vi "Marker Draw and Commands Loop.vi"(4 "Cursor Options":T1={"font"={"Font Name"="Arial", "Size"=15, "Strikeout?"=FALSE, "Italic?"=FALSE, "Underline?"=FALSE, "Outline?"=FALSE, "Shadow?"=FALSE, "Bold?"=FALSE}, "size"=2, "Timestamp"=enum."at BOTTOM", "Vertical Line?"=TRUE, "Horizontal Line?"=TRUE, "alignment(left, top)"={"horizontal"=enum."left", "vertical"=enum."center"}, "TextFormat"=" %3$s\\n %2$.2f", "time format (%H:%M:%S)"="%I:%M:%S %p"} {"size" min=1 max=50}, 6 "Enable Cursors":bool, 9 "Markers":T2[](array[typedef]), 10 "XY Graph":refnum<vi>, 11 "Options":T4={"Color"=16723218, "pen"={"Width"=2, "Style"=enum."Solid"}, "font"={"Font Name"="Arial", "Size"=14, "Strikeout?"=FALSE, "Italic?"=FALSE, "Underline?"=FALSE, "Outline?"=FALSE, "Shadow?"=FALSE, "Bold?"=FALSE, "FontColor"=6908265}, "caption"="Click to set a point marker"}) -> ()   [LabVIEW 2014, in "Graph Extensions.lvlib"]
doc: "This draw loop is the command processor thread and redraw thread to handle the events from the UI. It can be started anywhere with a reference to the graph. Markers work only when the graph palette tool is in cursor mode, as it replaces that mode since Graph extensions have their own improved cursors/markers, that mode is not needed. \n\n<B>Options</B> can be changed by the user using the right click menu with the markers.\n<B>Markers</B> input can be used to initialize a known set of markers (eitehr loaded from disk or programmatically created)\n\n<B>Cursers Enabled</B> activates the other graph extension (cursors) when usual mouse move occurs."
uses:
  Graph Extensions.lvlib
  controls/MarkerInfo.ctl
  <vilib>/Utility/miscctls.llb/LVPoint32TypeDef.ctl
  controls/markerType.ctl
  controls/commands.ctl
  controls/GraphExt-Cmds.ctl
  controls/cmd_options.ctl
  controls/Simple Global for Marker Options.vi
  controls/MarkerOptions.ctl
  controls/CursorOptions.ctl
panel:
  in  "stop":bool
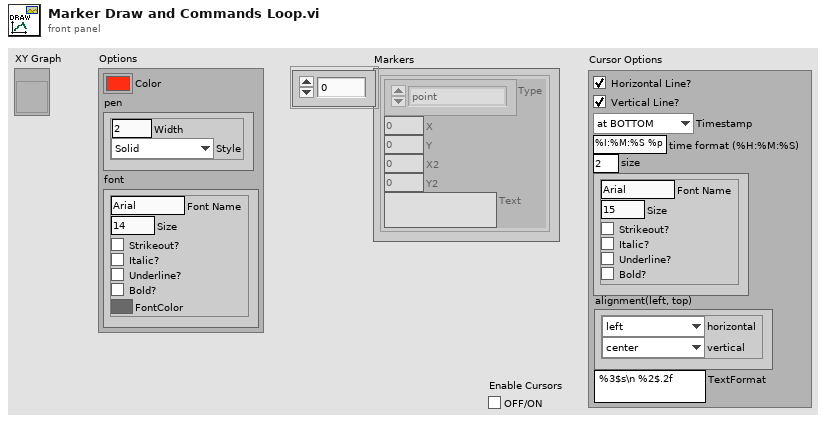
[diagram p1: front panel]
types:
  T1 = typedef "Graph Extensions.lvlib/CursorOptions.ctl" = cluster{"font":cluster{"Font Name":string, "Size":i16, "Strikeout?":bool, "Italic?":bool, "Underline?":bool, "Outline?":bool, "Shadow?":bool, "Bold?":bool}, "size":i16, "Timestamp":enum16{"at TOP", "at BOTTOM", "none"}, "Vertical Line?":bool, "Horizontal Line?":bool, "alignment(left, top)":cluster{"horizontal":enum16{"left", "center", "right"}, "vertical":enum16{"top", "center", "bottom"}}, "TextFormat":string, "time format (%H:%M:%S)":string}
  T2 = typedef "Graph Extensions.lvlib/MarkerInfo.ctl" = cluster{"Type":T3, "X":dbl, "Y":dbl, "X2":dbl, "Y2":dbl, "Text":string}
  T3 = typedef "Graph Extensions.lvlib/markerType.ctl" = enum16{"point", "arrow", "horiz", "vert", "vert range", "horiz range", "box"}
  T4 = typedef "Graph Extensions.lvlib/MarkerOptions.ctl" = cluster{"Color":u32, "pen":cluster{"Width":u16, "Style":enum32{"Solid", "Dash", "Dot", "DashDot", "DashDotDot"}}, "font":cluster{"Font Name":string, "Size":i16, "Strikeout?":bool, "Italic?":bool, "Underline?":bool, "Outline?":bool, "Shadow?":bool, "Bold?":bool, "FontColor":u32}, "caption":string}
  T5 = typedef "Graph Extensions.lvlib/commands.ctl" = enum16{"up", "options", "click", "move", "type", "redraw", "edited", "exit"}
  T6 = typedef "LVPoint32TypeDef.ctl" = cluster{"Horizontal":i32, "Vertical":i32}
  T7 = cluster{"cmd":T5, "Type":T3, "Coords":T6, "Active Tool":i32, "mode":enum16{"drag", "none"}}
  T8 = typedef "Graph Extensions.lvlib/GraphExt-Cmds.ctl" = cluster{"cmd":T5, "Type":T3, "Coords":T6, "text":string}
  T9 = typedef "Graph Extensions.lvlib/cmd_options.ctl" = cluster{"Marker Color":u32, "Style":enum32{"Solid", "Dash", "Dot", "DashDot", "DashDotDot"}, "Width":u16, "Size":i16, "Color":u32}
  T10 = typedef "LVRectTypeDef.ctl" = cluster{"Left":i16, "Top":i16, "Right":i16, "Bottom":i16}
  T11 = enum32{"Solid", "Dash", "Dot", "DashDot", "DashDotDot"}
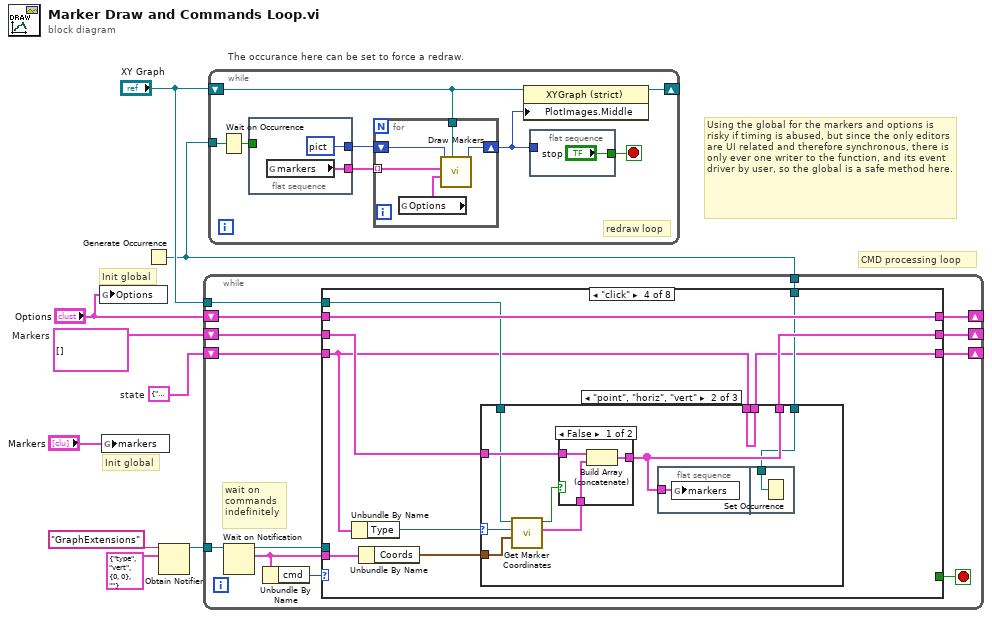
[diagram p0: block diagram]
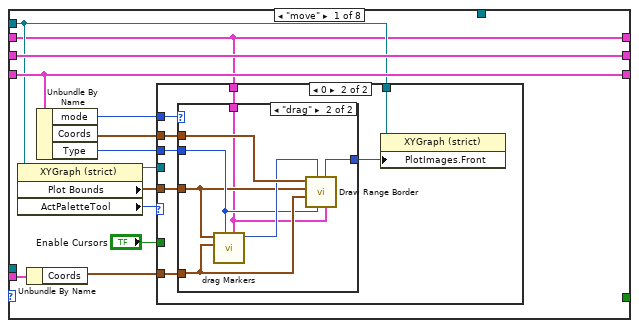
[diagram p2: hidden frame]
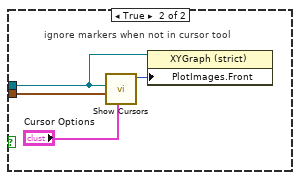
[diagram p4: hidden frame]
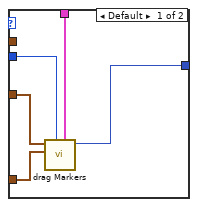
[diagram p5: hidden frame]
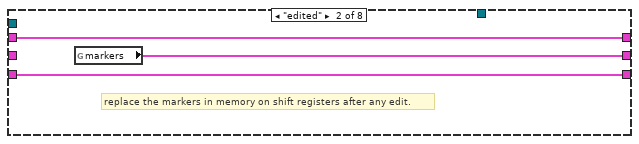
[diagram p6: hidden frame]
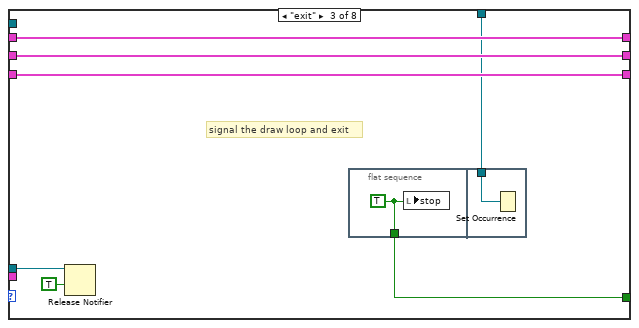
[diagram p7: hidden frame]
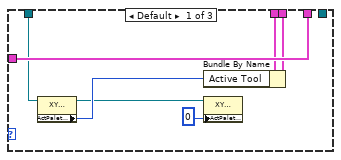
[diagram p8: hidden frame]
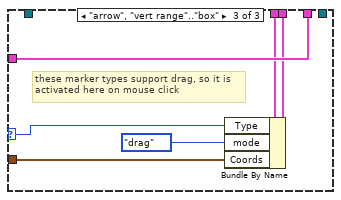
[diagram p10: hidden frame]
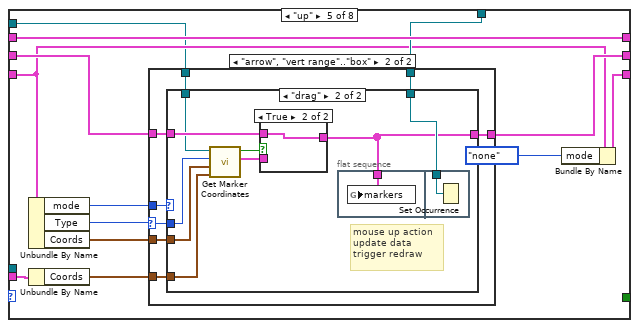
[diagram p11: hidden frame]
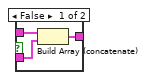
[diagram p14: hidden frame]
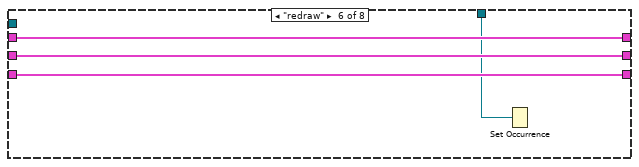
[diagram p15: hidden frame]
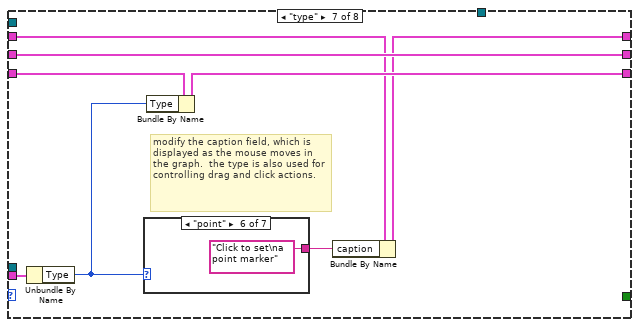
[diagram p16: hidden frame]
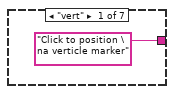
[diagram p17: hidden frame]
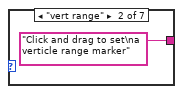
[diagram p18: hidden frame]
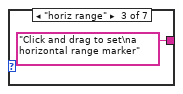
[diagram p19: hidden frame]
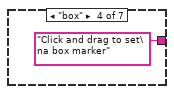
[diagram p20: hidden frame]
diagram:
  w5 = T7 {"cmd"=enum."click", "Type"=enum."point", "Coords"={"Horizontal"=0, "Vertical"=0}, "Active Tool"=0, "mode"=enum."none"}  # state
  w4 = T2[] []  # Markers
  # "Init global"
  # "CMD processing loop"
  # "Using the global for the markers and options is risky if timing is abused, but since the only editors are UI related and therefore synchronous, there is only ever one writer to the function, and its event driver by user, so the global is a safe method here."
  # "Init global"
  # "The occurance here can be set to force a redraw."
  n1 = global write "Simple Global for Marker Options.vi" "Options"("Options") -> ()
  n2 = global write "Simple Global for Marker Options.vi" "markers"("Markers") -> ()
  n3 = Generate Occurrence() -> (w3:refnum<k4>)
  n4 = Obtain Notifier(name (unnamed)="GraphExtensions", notification data type=T8 {"cmd"=enum."type", "Type"=enum."vert", "Coords"={"Horizontal"=0, "Vertical"=0}, "text"=""}) -> (notifier out=w8:refnum<notifier>)  [unwired: 2 in, 2 out]
  n5 = while {
    tunnel: w8 -> [w22]
    shift-right: [w18] -> _
    shift-left: "Options" -> [w19]
    shift-right: [w17] -> _
    shift-left: w4 -> [w16]
    shift-right: [w15] -> _
    shift-left: w5 -> [w14]
    tunnel: w3 -> [w13]
    tunnel: "XY Graph" -> [w12]
    stop <- w11 stop-if-true
    # "wait on\ncommands\nindefinitely"
    n6 = Wait on Notification(notifier=w22) -> (notifier out=w10:refnum<notifier>, notification=w21:T8)  [unwired: 3 in, 2 out]
    n7 = Unbundle By Name(w21) -> ("cmd"=w20:T5)
    n8 = case shown="\"click\"" w20 {
      tunnel: w19 -> [w26 w65 w72 w84 w125 w152 w156 w176]
      tunnel: w21 -> [w35 _ _ w83 w124 _ w161 w181]
      tunnel: [w26 w65 w72 w84 w125 w152 w155 w171] -> w18
      tunnel: [w34 w63 w71 w82 w118 w154 w162 w183] -> w17
      tunnel: w16 -> [w34 _ w71 w78 w119 w154 w162 w183]
      tunnel: [w33 w64 w70 w79 w115 w153 w159 w182] -> w15
      tunnel: w14 -> [w33 w64 w70 w77 w116 w153 w160 w182]
      tunnel: w13 -> [_ _ w68 w81 w117 w151 _ w170]
      tunnel: w12 -> [w28 _ _ w80 w113 _ _ _]
      tunnel: [_ _ w69 _ _ _ _ _] -> w11
      tunnel: w10 -> [_ _ w67 _ _ _ _ _]
      frame "move" {
        n9 = property on="Property Node" class="XYGraph (strict)"(reference=w28) -> (reference out=w24:refnum<vi>, "Plot Bounds"=w27:T10, "ActPaletteTool"=w25:i32)  [unwired: 1 in, 1 out]
        n10 = Unbundle By Name(w35) -> ("Coords"=w29:T6)
        n11 = Unbundle By Name(w33) -> ("mode"=w31:enum16{"drag", "none"}, "Coords"=w32:T6, "Type"=w30:T3)
        n12 = case shown="0" w25 {
          tunnel: w32 -> [_ w50]
          tunnel: w31 -> [_ w48]
          tunnel: w30 -> [_ w47]
          tunnel: w29 -> [w37 w46]
          tunnel: w28 -> [_ w45]
          tunnel: w27 -> [_ w44]
          tunnel: w26 -> [_ w43]
          tunnel: w24 -> [w38 _]
          tunnel: "Enable Cursors" -> [w36 _]
          frame Default {
            n13 = case shown="False" w36 {
              tunnel: w38 -> [_ w40]
              tunnel: w37 -> [_ w39]
              frame False {
              }
              frame True {
                # "ignore markers when not in cursor tool"
                n14 = call "Show Cursors.vi"("Cursor Options"="Cursor Options", "Coords"=w39, "XY Graph"=w40) -> ("output picture"=w42:picture)  [unwired: 7 in, 1 out]
                n15 = property on="Property Node" class="XYGraph (strict)"(reference=w40, "PlotImages.Front"=w42) -> ()  [unwired: 1 in, 2 out]
              }
            }
          }
          frame 0 {
            n16 = case shown="\"drag\"" w48 {
              tunnel: w50 -> [_ w62]
              tunnel: [w55 w61] -> w49
              tunnel: w43 -> [w54 w56]
              tunnel: w47 -> [w53 w58]
              tunnel: w46 -> [w52 w59]
              tunnel: w44 -> [w51 w57]
              frame Default {
                n17 = call "drag Markers.vi"("Marker Options"=w54, "Type"=w53, "Coords"=w52, "Plot Area Bounds"=w51) -> ("new picture"=w55:picture)  [unwired: 7 in]
              }
              frame "drag" {
                n18 = call "drag Markers.vi"("Marker Options"=w56, "Type"=w58, "Coords"=w59, "Plot Area Bounds"=w57) -> ("new picture"=w60:picture)  [unwired: 7 in]
                n19 = call "Draw Range Border.vi"("Marker Options"=w56, "Type"=w58, "picture"=w60, "end Coords"=w59, "Plot Bounds"=w57, "Start Coords"=w62) -> ("new picture"=w61:picture)  [unwired: 5 in]
              }
            }
            n20 = property on="Property Node" class="XYGraph (strict)"(reference=w45, "PlotImages.Front"=w49) -> ()  [unwired: 1 in, 2 out]
          }
        }
      }
      frame "edited" {
        # "replace the markers in memory on shift registers after any edit."
        n21 = global read "Simple Global for Marker Options.vi" "markers"() -> (w63:T2[])
      }
      frame "exit" {
        # "signal the draw loop and exit"
        n22 = Release Notifier(notifier=w67, force destroy? (F)=TRUE) -> ()  [unwired: 1 in, 3 out]
        n23 = flat-sequence {
          tunnel: [w73] -> w69
          tunnel: w68 -> [w74]
          frame #0 {
            w73 = TRUE
            n24 = local write "stop"(w73) -> ()
          }
          frame #1 {
            n25 = Set Occurrence(w74) -> ()
          }
        }
      }
      frame "click" {
        n26 = Unbundle By Name(w77) -> ("Type"=w76:T3)
        n27 = Unbundle By Name(w83) -> ("Coords"=w75:T6)
        n28 = case shown="\"point\", \"horiz\", \"vert\"" w76 {
          selector: w76 -> [_ w97 w108]
          tunnel: w78 -> [w91 w100 w112]
          tunnel: [w91 w99 w112] -> w82
          tunnel: w81 -> [_ w96 _]
          tunnel: w80 -> [w90 w95 _]
          tunnel: w77 -> [w89 w98 w111]
          tunnel: [w88 w98 w110] -> w79
          tunnel: w75 -> [_ w94 w107]
          frame Default {
            n29 = property class="XYGraph (strict)"(reference=w90) -> (reference out=w86:refnum<vi>, "ActPaletteTool"=w87:i32)  [unwired: 1 in, 1 out]
            n30 = Bundle By Name(cluster=w89, "Active Tool"=w87) -> (w88:T7)
            n31 = property class="XYGraph (strict)"(reference=w86, "ActPaletteTool"=0 ("Palette:Active Tool")) -> ()  [unwired: 1 in, 2 out]
          }
          frame "point", "horiz", "vert" {
            n32 = call "Get Marker Coordinates.vi"("Point32"=w94, "Type"=w97, "XYGraph in"=w95) -> ("Markers"=w92:T2, "Cancelled"=w93:bool)  [unwired: 7 in]
            n33 = case shown="False" w93 {
              tunnel: w100 -> [w103 w104]
              tunnel: w92 -> [w102 _]
              tunnel: [w101 w104] -> w99
              frame False {
                n34 = Build Array (concatenate)(w103, w102) -> (w101:T2[])
              }
              frame True {
              }
            }
            n35 = flat-sequence {
              tunnel: w99 -> [w105]
              tunnel: w96 -> [w106]
              frame #0 {
                n36 = global write "Simple Global for Marker Options.vi" "markers"(w105) -> ()
              }
              frame #1 {
                n37 = Set Occurrence(w106) -> ()
              }
            }
          }
          frame "arrow", "vert range".."box" {
            # "these marker types support drag, so it is\nactivated here on mouse click"
            n38 = Bundle By Name(cluster=w111, "Type"=w108, "mode"=enum16{"drag", "none"}."drag", "Coords"=w107) -> (w110:T7)
          }
        }
      }
      frame "up" {
        n39 = Unbundle By Name(w116) -> ("mode"=w120:enum16{"drag", "none"}, "Type"=w123:T3, "Coords"=w122:T6)
        n40 = Unbundle By Name(w124) -> ("Coords"=w121:T6)
        n41 = case shown="\"arrow\", \"vert range\"..\"box\"" w123 {
          selector: w123 -> [_ w133]
          tunnel: w122 -> [_ w129]
          tunnel: w121 -> [_ w130]
          tunnel: w120 -> [_ w134]
          tunnel: w119 -> [w126 w132]
          tunnel: [w126 w131] -> w118
          tunnel: w117 -> [_ w128]
          tunnel: w113 -> [_ w127]
          frame Default {
            # "mouse up is not supported for these marker types\nor is not needed, since they are single click"
          }
          frame "arrow", "vert range".."box" {
            n42 = case shown="\"drag\"" w134 {
              tunnel: w133 -> [_ w141]
              tunnel: w132 -> [w135 w144]
              tunnel: [w135 w142] -> w131
              tunnel: w130 -> [_ w136]
              tunnel: w129 -> [_ w140]
              tunnel: w128 -> [_ w143]
              tunnel: w127 -> [_ w139]
              frame Default {
                # "if drag mode was not already active\nthen the up event can be ignored."
              }
              frame "drag" {
                # "mouse up action\nupdate data\ntrigger redraw"
                n43 = call "Get Marker Coordinates.vi"("Coords 2"=w136, "Point32"=w140, "Type"=w141, "XYGraph in"=w139) -> ("Markers"=w137:T2, "Cancelled"=w138:bool)  [unwired: 6 in]
                n44 = case shown="True" w138 {
                  tunnel: w144 -> [w147 w148]
                  tunnel: [w146 w148] -> w142
                  tunnel: w137 -> [w145 _]
                  frame False {
                    n45 = Build Array (concatenate)(w147, w145) -> (w146:T2[])
                  }
                  frame True {
                  }
                }
                n46 = flat-sequence {
                  tunnel: w142 -> [w149]
                  tunnel: w143 -> [w150]
                  frame #0 {
                    n47 = global write "Simple Global for Marker Options.vi" "markers"(w149) -> ()
                  }
                  frame #1 {
                    n48 = Set Occurrence(w150) -> ()
                  }
                }
              }
            }
          }
        }
        n49 = Bundle By Name(cluster=w116, "mode"=enum16{"drag", "none"}."none") -> (w115:T7)
      }
      frame "redraw" {
        n50 = Set Occurrence(w151) -> ()
      }
      frame "type" {
        # "modify the caption field, which is displayed as the mouse moves in the graph.  the type is also used for controlling drag and click actions."
        n51 = Unbundle By Name(w161) -> ("Type"=w158:T3)
        n52 = case shown="\"point\"" w158 {
          tunnel: ["Click to position \na verticle marker" ("Text") "Click and drag to set\na verticle range marker" ("Text") "Click and drag to set\na horizontal range marker" ("Text") "Click and drag to set\na box marker" ("Text") "Click and drag to draw an arrow" ("Text") "Click to set\na point marker" ("Text") "Click to position \na horizontal marker" ("Text")] -> w157
          frame "vert" {
          }
          frame "vert range" {
          }
          frame "horiz range" {
          }
          frame "box" {
          }
          frame "arrow" {
          }
          frame "point" {
          }
          frame "horiz" {
          }
        }
        n53 = Bundle By Name(cluster=w160, "Type"=w158) -> (w159:T7)
        n54 = Bundle By Name(cluster=w156, "caption"=w157) -> (w155:T4)
      }
      frame "options" {
        # "updates the options for drawing"
        # "Only writer to this global data"
        n55 = Unbundle By Name(w181) -> ("text"=w180:string)
        n56 = Unflatten From String(type=T9 {"Marker Color"=0, "Style"=enum."Solid", "Width"=0, "Size"=0, "Color"=0} ("cluster"), binary string=w180) -> (value=w179:T9)  [unwired: 3 in, 2 out]
        n57 = Unbundle By Name(w179) -> ("Marker Color"=w177:u32, "Style"=w175:T11, "Width"=w174:u16, "Size"=w173:i16, "Color"=w172:u32)
        n58 = Bundle By Name(cluster=w176, "Color"=w177, "pen.Style"=w175, "pen.Width"=w174, "font.Size"=w173, "font.FontColor"=w172) -> (w171:T4)
        n59 = flat-sequence {
          tunnel: w171 -> [w184]
          tunnel: w170 -> [w185]
          frame #0 {
            n60 = global write "Simple Global for Marker Options.vi" "Options"(w184) -> ()
          }
          frame #1 {
            n61 = Set Occurrence(w185) -> ()
          }
        }
      }
    }
  }
  n62 = while {
    shift-right: [w188] -> _
    shift-left: "XY Graph" -> [w187]
    tunnel: w3 -> [w193]
    stop <- w189 stop-if-true
    # "redraw loop"
    n63 = Wait on Occurrence(2:w193) -> (0:w190:bool)  [unwired: 2 in]
    n64 = flat-sequence {
      tunnel: [w195] -> w192
      tunnel: [picture data[5B] ("new picture")] -> w191
      tunnel: w190 -> [_]
      frame #0 {
        n65 = global read "Simple Global for Marker Options.vi" "markers"() -> (w195:T2[])
      }
    }
    n66 = for {
      tunnel: w192 -> [w201] mode=indexing
      shift-right: [w199] -> w186
      shift-left: w191 -> [w200]
      tunnel: w187 -> [w198]
      n67 = global read "Simple Global for Marker Options.vi" "Options"() -> (w197:T4)
      n68 = call "Draw Markers.vi"("XYGraph in"=w198, "Marker Options"=w197, "Marker"=w201, "picture"=w200) -> ("new picture"=w199:picture)  [unwired: 7 in]
    }
    n69 = property class="XYGraph (strict)"(reference=w187, "PlotImages.Middle"=w186) -> (reference out=w188:refnum<vi>)  [unwired: 1 in, 1 out]
    n70 = flat-sequence {
      tunnel: ["stop"] -> w189
      tunnel: w186 -> [_]
      frame #0 {
      }
    }
  }
